vi "2 Helper - compute fake polar plot.vi"() -> ()   [LabVIEW 2011]
panel:
  out "Waveform Graph":dbl[](graph)
  out "Lookup Table":dbl[](array[numeric])
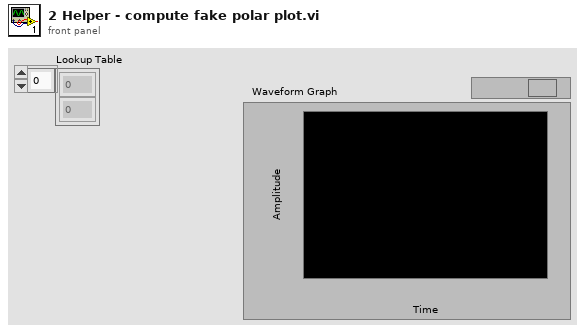
[diagram p1: front panel]
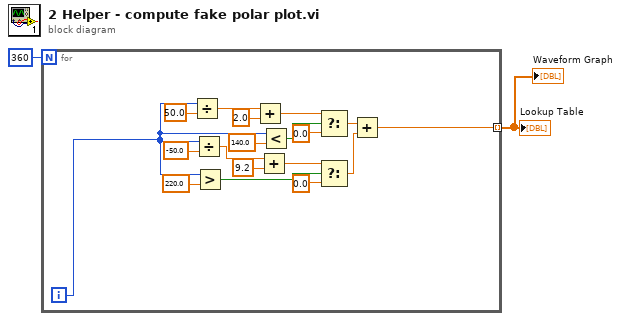
[diagram p0: block diagram]
diagram:
  n1 = for {
    N: 360 -> [_]
    tunnel: [w3] -> w1 mode=indexing
    i -> [w4]
    n2 = Divide(x=w4, y=50.0) -> (x/y=w12:dbl)
    n3 = Divide(x=w4, y=-50.0) -> (x/y=w7:dbl)
    n4 = Greater?(x=w4, y=220.0) -> (0:w15:bool)
    n5 = Add(x=w12, y=2.0) -> (x+y=w13:dbl)
    n6 = Add(x=w7, y=9.2) -> (x+y=w5:dbl)
    n7 = Less?(x=w4, y=140.0) -> (x < y?=w19:bool)
    n8 = Select(t=w13, s=w19, f=0.0) -> (s? t:f=w10:dbl)
    n9 = Select(t=w5, s=w15, f=0.0) -> (s? t:f=w9:dbl)
    n10 = Add(x=w10, y=w9) -> (x+y=w3:dbl)
  }
  "Lookup Table" <- w1
  "Waveform Graph" <- w1
